vi "Reset Swerve.vi"(8 "error in":errorcluster, 10 "Encoder Offset":i32=-3302, 11 "Enum":T1=enum."Swerve 1") -> (0 "error out":errorcluster, 3 "Final Offset":dbl=3306.0)   [LabVIEW 2016]
uses:
  Refname/Motors.ctl
  Main/Robot Global Data.vi
  Refname/Refname to String (Motors).vi
panel:
  in  "Time Target (s)":dbl=0.5
  in  "Tolerance":dbl=5.0 format="%#_13g"
  out "CAN.Device Number":u8=2
  in  "PID gains":T2={"proportional gain (Kc)"=5.0, "integral time (Ti, min)"=0.032, "derivative time (Td, min)"=0.0} {"derivative time (Td, min)" format="%.3f"; "integral time (Ti, min)" format="%.8f"; "proportional gain (Kc)" format="%.8f"}
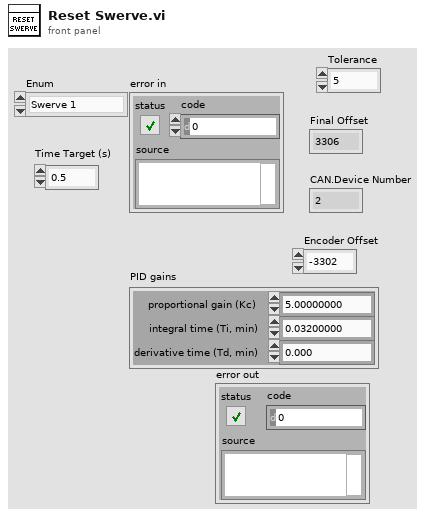
[diagram p1: front panel]
types:
  T1 = typedef "Motors.ctl" = enum16{"Wheel 1", "Swerve 1", "Wheel 2", "Swerve 2", "Wheel 3", "Swerve 3", "Wheel 4", "Swerve 4"}
  T2 = cluster{"proportional gain (Kc)":dbl, "integral time (Ti, min)":dbl, "derivative time (Td, min)":dbl}
  T3 = typedef "WPI_MotorControlDeviceRef.ctl" = cluster{"DeviceStatus":errorcluster, "Type":T4, "PWM":cluster{"PWM Channel":T5, "DeadBand":T6}, "CAN":cluster{"Device Number":u8, "SetOutput VI Ref":variant, "GetOutput VI Ref":variant, "Enable VI Ref":variant, "Disable VI Ref":variant, "Data":variant}, "Invert":bool}
  T4 = typedef "WPI_MotorControlType.ctl" = enum16{"PWM", "CAN"}
  T5 = typedef "FPGA_DIOPWMChannel.ctl" = enum8{"PWM 0", "PWM 1", "PWM 2", "PWM 3", "PWM 4", "PWM 5", "PWM 6", "PWM 7", "PWM 8", "PWM 9", "PWM MXP 0", "PWM MXP 1", "PWM MXP 2", "PWM MXP 3", "PWM MXP 4", "PWM MXP 5", "PWM MXP 6", "PWM MXP 7", "PWM MXP 8", "PWM MXP 9", "Invalid"}
  T6 = typedef "WPI_PWMDeadband.ctl" = cluster{"Name":string, "maxPositivePwm":i32, "minPositivePwm":i32, "centerPwm":i32, "maxNegativePwm":i32, "minNegativePwm":i32, "angularRange":u16}
  T7 = typedef "WPI_CANTalonSRX_GlobalStatus.ctl" = cluster{"Applied Throttle":dbl, "Module Enabled":bool, "CAN Error":errorcluster, "Closed Loop Error":dbl, "Forward Limit Switch Closed":bool, "Reverse Limit Switch Closed":bool, "Sensor Position":dbl, "Sensor Velocity":dbl, "Current":dbl, "Sticky Fault - Over Temp":bool, "Sticky Fault - Under Voltage":bool, "Sticky Fault - Forward Limit":bool, "Sticky Fault - Reverse Limit":bool, "Sticky Fault - Forward Soft Limit":bool, "Sticky Fault - Reverse Soft Limit":bool, "Brake is Enabled":bool, "Encoder Position":dbl, "Encoder Velocity":dbl, "Encoder Index Count":dbl, "Encoder A Pin State":bool, "Encoder B Pin State":bool, "Encoder Index Pin State":bool, "Analog In":dbl, "Analog In Velocity":dbl, "Temperature (C)":dbl, "Battery Voltage":dbl, "Control 5 Is Supported":bool, "Current Profile Slot Select":dbl, "Pos Div 8":bool, "Vel Div 4":bool, "Pulse Width Position":i32, "Pulse Width Velocity":i32, "Pulse Width Rise To Rise (us)":i32, "Pulse Width Rise To Fall (us)":i32, "Mot Prof Active Is Under Run":bool, "Mot Prof Active Has Under Run":bool, "Mot Prof Active Is Last":bool, "Mot Prof Active Velocity Only":bool, "Mot Prof Active Is Valid":bool, "Mot Prof Buffer Is Full":bool, "Mot Prof Active Profile Slot Select":i32, "Mot Prof NextID":i32, "Mot Prof Count":i32, "Mot Prof Active Velocity":dbl, "Mot Prof Active Position":dbl, "Mot Prof Output Enable":i32}
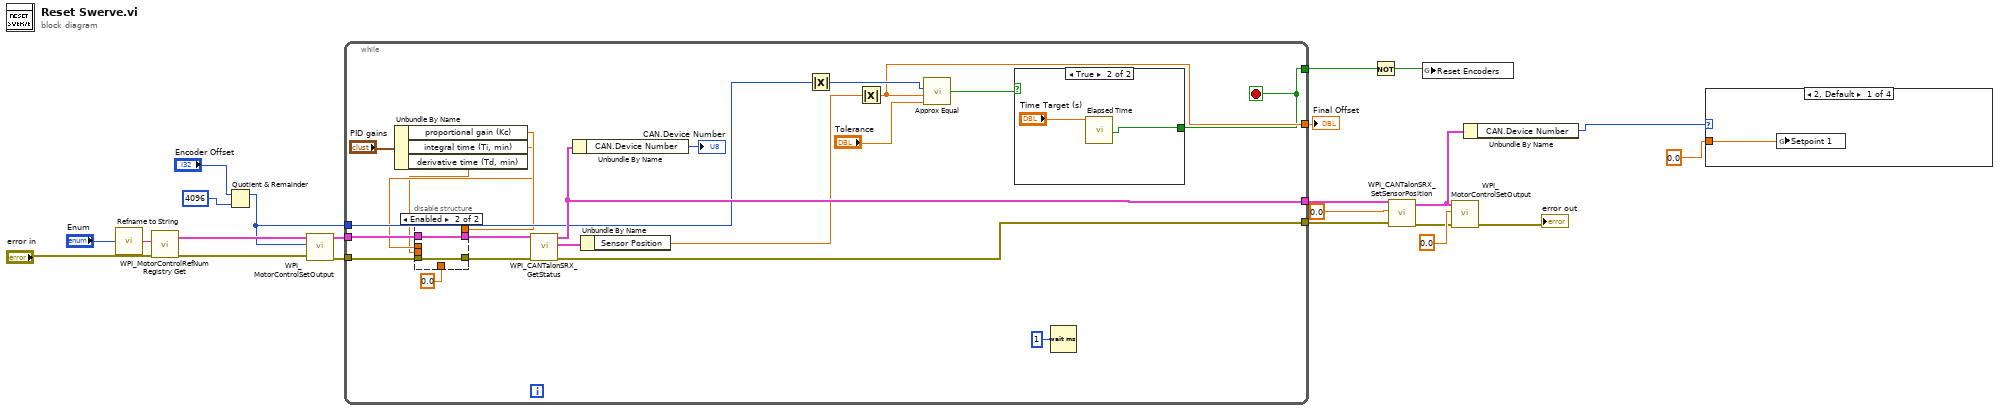
[diagram p0: block diagram]
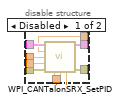
[diagram p2: hidden frame]
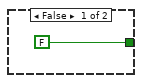
[diagram p3: hidden frame]
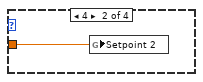
[diagram p4: hidden frame]
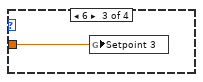
[diagram p5: hidden frame]
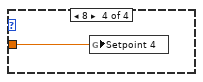
[diagram p6: hidden frame]
diagram:
  n1 = call-poly "Refname to String.vi"("Enum"="Enum") -> ("String"=w21:string)
  n2 = call <vilib>:"WPI_MotorControlRefNum Registry Get.vi"("error in (no error)"="error in", "refnum name"=w21) -> ("error out"=w18:errorcluster, "MotorControlDevRef"=w17:T3)  [unwired: 8 in]
  n3 = Quotient & Remainder(x="Encoder Offset", y=4096) -> (x-y*floor(x/y)=w12:i32)  [unwired: 1 out]
  n4 = call <vilib>:"WPI_MotorControlSetOutput.vi"("error in (no error)"=w18, "Output"=w12, "MotorControlDevRef"=w17) -> ("error out"=w15:errorcluster, "MotorControlDevRef"=w16:T3)  [unwired: 6 in, 1 out]
  n5 = while {
    tunnel: w16 -> [w35]
    tunnel: w15 -> [w33]
    tunnel: [w40] -> w10
    tunnel: w12 -> [w36]
    tunnel: [w37] -> w11
    tunnel: [w25] -> w1
    tunnel: [w24] -> w8
    stop <- w24 stop-if-true
    n6 = Unbundle By Name("PID gains") -> ("proportional gain (Kc)"=w31:dbl, "integral time (Ti, min)"=w30:dbl, "derivative time (Td, min)"=w29:dbl)
    n7 = disable-structure shown="Enabled" {
      disable-tunnel: w35 -> [w51 w53]
      disable-tunnel: [w50 w52] -> w34
      disable-tunnel: w33 -> [w49 w52]
      disable-tunnel: w31 -> [w48 _]
      disable-tunnel: w30 -> [w47 _]
      disable-tunnel: w29 -> [w46 _]
      disable-tunnel: 0.0 ("Output") -> [w45 _]
      disable-tunnel: [w44 w53] -> w27
      frame Disabled {
        n8 = call <vilib>:"WPI_CANTalonSRX_SetPID.vi"("CAN Talon SRX Ref"=w51, "P"=w48, "I"=w47, "D"=w46, "error in (no error)"=w49, "F"=w45, "I Zone"=w45, "Ramp Rate"=w45) -> ("CAN Talon SRX Ref"=w44:T3, "error out"=w50:errorcluster)  [unwired: 6 in]
      }
      frame Enabled {
      }
    }
    n9 = call <vilib>:"WPI_CANTalonSRX_GetStatus.vi"("error in (no error)"=w34, "CAN Talon SRX Ref"=w27) -> ("error out"=w40:errorcluster, "Talon SRX Status"=w41:T7, "CAN Talon SRX Ref"=w37:T3)  [unwired: 7 in]
    n10 = Unbundle By Name(w37) -> ("CAN.Device Number"=→"CAN.Device Number":u8)
    n11 = Unbundle By Name(w41) -> ("Sensor Position"=w23:dbl)
    n12 = Absolute Value(x=w36) -> (abs(x)=w26:i32)
    n13 = Absolute Value(x=w23) -> (abs(x)=w25:dbl)
    n14 = call "Approx Equal.vi"("Tolerance"="Tolerance", "b"=w25, "a"=w26) -> ("a == b?"=w38:bool)  [unwired: 1 in]
    n15 = case shown="True" w38 {
      tunnel: [FALSE w55] -> w24
      frame False {
      }
      frame True {
        n16 = call "Elapsed Time"("Time Target (s)"="Time Target (s)") -> ("Time has Elapsed"=w55:bool)  [unwired: 11 in, 7 out]
      }
    }
    n17 = Wait (ms)(milliseconds to wait=u32 1) -> ()  [unwired: 1 out]
  }
  "Final Offset" <- w1
  n18 = Not(x=w8) -> (.not. x?=w19:bool)
  n19 = call <vilib>:"WPI_CANTalonSRX_SetSensorPosition.vi"("error in (no error)"=w10, "New Sensor Position"=0.0, "CAN Talon SRX Ref"=w11) -> ("error out"=w6:errorcluster, "CAN Talon SRX Ref"=w3:T3)  [unwired: 7 in]
  n20 = global write "Robot Global Data.vi" "Reset Encoders"(w19) -> ()
  n21 = call <vilib>:"WPI_MotorControlSetOutput.vi"("error in (no error)"=w6, "Output"=0.0 ("New Sensor Position"), "MotorControlDevRef"=w3) -> ("error out"=→"error out":errorcluster)  [unwired: 6 in, 2 out]
  n22 = Unbundle By Name(w3) -> ("CAN.Device Number"=w2:u8)
  n23 = case shown="2, Default" w2 {
    tunnel: 0.0 ("New Sensor Position") -> [w57 w58 w59 w60]
    frame 2, Default {
      n24 = global write "Robot Global Data.vi" "Setpoint 1"(w57) -> ()
    }
    frame 4 {
      n25 = global write "Robot Global Data.vi" "Setpoint 2"(w58) -> ()
    }
    frame 6 {
      n26 = global write "Robot Global Data.vi" "Setpoint 3"(w59) -> ()
    }
    frame 8 {
      n27 = global write "Robot Global Data.vi" "Setpoint 4"(w60) -> ()
    }
  }
